vi "Construct Aggregate.vi"(8 "error in (no error)":errorcluster, 9 "Reflection.Tests.lvlib:Child.lvclass":refnum<class "Child.lvclass">, 10 "Reflection.Tests.lvlib:String.lvclass":refnum<class "String.lvclass">) -> (0 "error out":errorcluster, 3 "Aggregate out":refnum<class "Aggregate.lvclass">)   [LabVIEW 2017, in "Composition.Tests.lvlib" / "Aggregate.lvclass"]
uses:
  Aggregate.lvclass
  String/String.lvclass
  Child/Child.lvclass
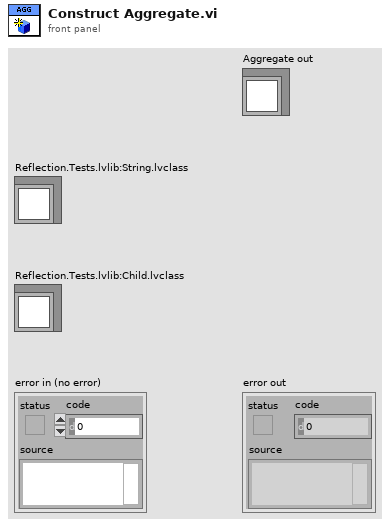
[diagram p1: front panel]
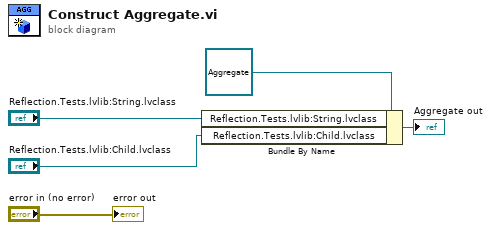
[diagram p0: block diagram]
diagram:
  n1 = Bundle By Name(cluster=refnum<class "Aggregate.lvclass"> refnum ("Aggregate in"), "Reflection.Tests.lvlib:String.lvclass"="Reflection.Tests.lvlib:String.lvclass", "Reflection.Tests.lvlib:Child.lvclass"="Reflection.Tests.lvlib:Child.lvclass") -> (→"Aggregate out":refnum<class "Aggregate.lvclass">)
  "error out" <- "error in (no error)"
